vi "LVProjectShortcut_RetrieveFileSelectionMode.vi"(8 "error in":errorcluster, 11 "Ctl Refnum":refnum<vi>) -> (0 "error out":errorcluster, 2 "Selection Mode":T1(ring))   [LabVIEW 2017, in "LVProject Shortcut.lvlib"]
doc: "Retrieves <b>Selection mode</b> as Object Tag of the control specified by <b>Ctl Refnum</b>."
uses:
  LVProject Shortcut.lvlib
  <vilib>/UserTags/UserTags.lvlib
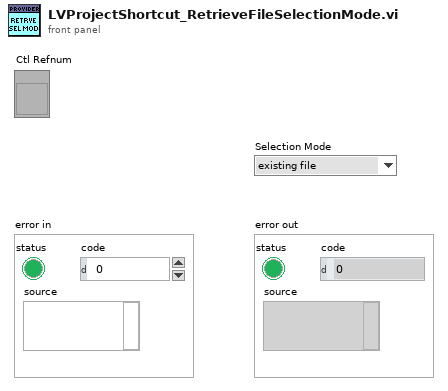
[diagram p1: front panel]
types:
  T1 = enum32{"existing file", "new file", "new or existing file", "existing dir", "new dir", "new or existing dir", "existing file (use LLBs)", "new file (use LLBs)", "new or existing file (use LLBs)", "new or existing file or directory (use LLBs)", "existing dir (use LLBs)", "new dir (use LLBs)", "new or existing dir (use LLBs)", "existing file or dir", "new file or dir", "new or existing file or dir", "existing file or dir (use LLBs)", "new file or dir (use LLBs)"}
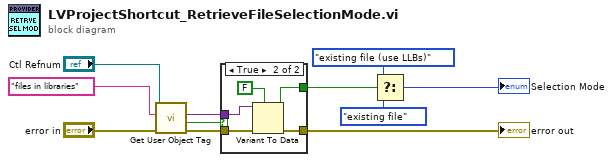
[diagram p0: block diagram]
diagram:
  n1 = call <vilib>:"Get User Object Tag.vi"("error in (no error)"="error in", "Tag Name"="files in libraries", "Generic Refnum"="Ctl Refnum") -> ("error out"=w7:errorcluster, "Was Tag Found?"=w5:bool, "Value"=w8:variant)  [unwired: 5 in, 1 out]
  n2 = case shown="True" w5 {
    tunnel: w8 -> [_ w17]
    tunnel: w7 -> [w12 w15]
    tunnel: [_ w14] -> w2
    tunnel: [w12 w13] -> w6
    frame False {
    }
    frame True {
      n3 = Variant To Data(error in=w15, type=FALSE, Variant=w17) -> (data=w14:bool, error out=w13:errorcluster)
    }
  }
  "error out" <- w6
  n4 = Select(t=T1."existing file (use LLBs)" ("Browse Options:Selection Mode"), s=w2, f=T1."existing file" ("Browse Options:Selection Mode")) -> (s? t:f=→"Selection Mode":T1)
